vi "Post-Build Action.vi"(5 "Files Generated by Build":path[](array[path]) caption="Fichiers générés par la construction", 6 "Top Level/Always Included VIs":path[](array[path]) caption="VIs Niveau principal/Toujours inclus", 7 "Destination Path":path caption="Chemin de destination", 8 "error in (no error)":errorcluster caption="entrée d'erreur (pas d'erreur)", 9 "Target Name":string caption="Nom de la cible", 10 "Build Specification Name":string caption="Nom de la spécification de construction", 11 "Project Path":path caption="Chemin du projet") -> (0 "error out":errorcluster caption="sortie d'erreur")   [LabVIEW 2020]
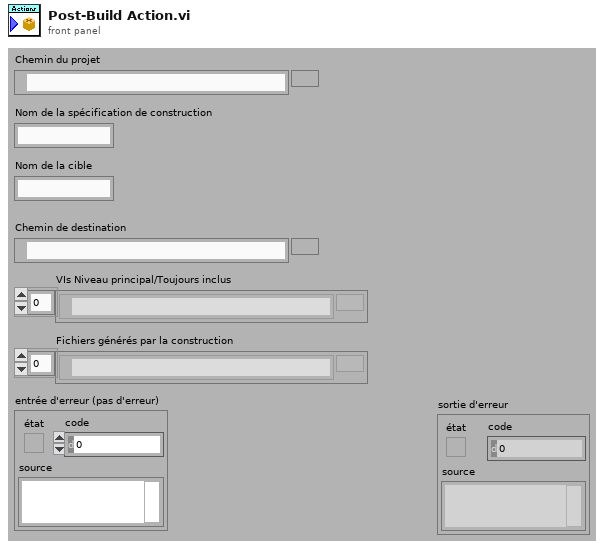
[diagram p1: front panel]
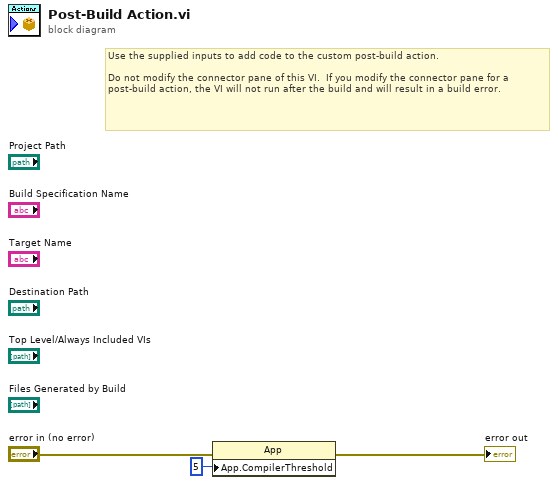
[diagram p0: block diagram]
diagram:
  # "Use the supplied inputs to add code to the custom post-build action.\n\nDo not modify the connector pane of this VI.  If you modify the connector pane for a post-build action, the VI will not run after the build and will result in a build error."
  n1 = property class="App"(error in="error in (no error)", "App.CompilerThreshold"=u32 5 ("Application:Seuil du compilateur")) -> (error out=→"error out":errorcluster)  [unwired: 1 in, 1 out]
